vi "Graph.vi"(8 "error in (no error)":errorcluster, 10 "notifier out":refnum<notifier>, 11 "State in":T1={"State"=enum."Idle", "Start Time"=timestamp(0 s since 1904-01-01), "Current Time"=timestamp(0 s since 1904-01-01), "First Iteration"=FALSE, "Data"={"D-O State"=enum."Off"}, "Process Name"="", "Output Error"=FALSE, "Log Started"=FALSE, "Cycle Period"=50.0, "Configuration"={"Valve Settings"={"D-O Settings"={"DAQmx Task Name"="", "Output Channel"=0, "Output Channel Names"=[]}, "VICI Electronic Actuator"={"VISA resource name"="", "Mode"=enum."Two Positions With Stops", "Simulated"=FALSE}}, "Valve Type"=enum."Digital Output Valve", "Time On (Sec)"=0.0, "Time Off (Sec)"=0.0, "Run?"=FALSE}} {"Configuration"."Valve Settings"."D-O Settings"."Output Channel" items=["Choose a Channel"]}) -> (0 "error out":errorcluster, 3 "State out":T1={"State"=enum."Idle", "Start Time"=timestamp(0 s since 1904-01-01), "Current Time"=timestamp(0 s since 1904-01-01), "First Iteration"=FALSE, "Data"={"D-O State"=enum."Off"}, "Process Name"="", "Output Error"=FALSE, "Log Started"=FALSE, "Cycle Period"=50.0, "Configuration"={"Valve Settings"={"D-O Settings"={"DAQmx Task Name"="", "Output Channel"=0, "Output Channel Names"=[]}, "VICI Electronic Actuator"={"VISA resource name"="", "Mode"=enum."Two Positions With Stops", "Simulated"=FALSE}}, "Valve Type"=enum."Digital Output Valve", "Time On (Sec)"=0.0, "Time Off (Sec)"=0.0, "Run?"=FALSE}} {"Configuration"."Valve Settings"."D-O Settings"."Output Channel" items=["Choose a Channel"]})   [LabVIEW 2018, in "D-O Module.lvlib" / "D-O Module Engine.lvlib"]
uses:
  D-O Module Engine.lvlib
  State Cluster.ctl
  State Enum.ctl
  Valve Clusters.ctl
  D-O Module Settings Cluster.ctl
  D-O Device Settings Cluster.ctl
  VICI Electronic Actuator/VICI Electronic Actuator Settings.ctl
  D-O Module.lvlib
  DIO Valve/VICI Electronic Actuator.lvlib
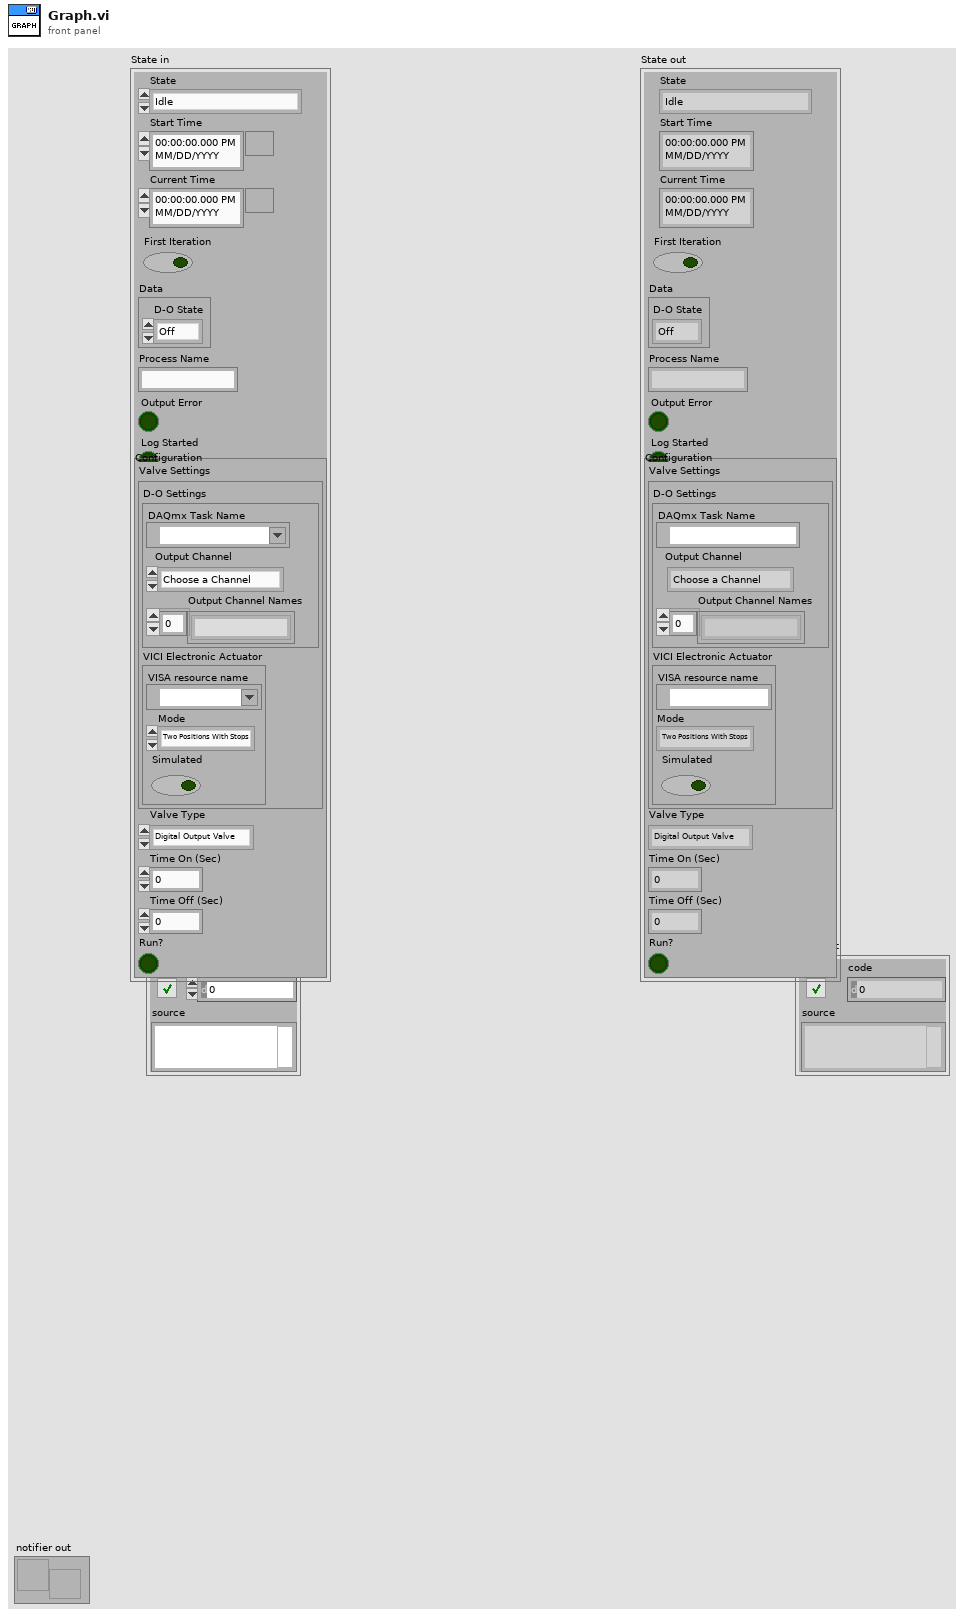
[diagram p1: front panel]
types:
  T1 = typedef "D-O Module.lvlib/D-O Module Engine.lvlib/State Cluster.ctl" = cluster{"State":T2, "Start Time":timestamp, "Current Time":timestamp, "First Iteration":bool, "Data":cluster{"D-O State":enum16{"Off", "On", "Not Initialized"}}, "Process Name":string, "Output Error":bool, "Log Started":bool, "Cycle Period":dbl, "Configuration":T3}
  T2 = typedef "D-O Module.lvlib/D-O Module Engine.lvlib/State Enum.ctl" = enum16{"Measuring", "Idle", "Paused"}
  T3 = typedef "D-O Module.lvlib/Valve Clusters.ctl" = cluster{"Valve Settings":T4, "Valve Type":enum16{"Default", "Digital Output Valve", "VICI Electronic Actuator"}, "Time On (Sec)":dbl, "Time Off (Sec)":dbl, "Run?":bool}
  T4 = typedef "D-O Module.lvlib/D-O Module Settings Cluster.ctl" = cluster{"D-O Settings":T5, "VICI Electronic Actuator":T6}
  T5 = typedef "D-O Module.lvlib/D-O Device Settings Cluster.ctl" = cluster{"DAQmx Task Name":refnum<k21>, "Output Channel":u16, "Output Channel Names":string[]}
  T6 = typedef "VICI Electronic Actuator.lvlib/VICI Electronic Actuator Settings.ctl" = cluster{"VISA resource name":refnum<visa-resource-name>, "Mode":enum16{"Two Positions With Stops", "Two Positions Without Stops", "Mutiposition"}, "Simulated":bool}
  T7 = cluster{"D-O State":enum16{"Off", "On", "Not Initialized"}}
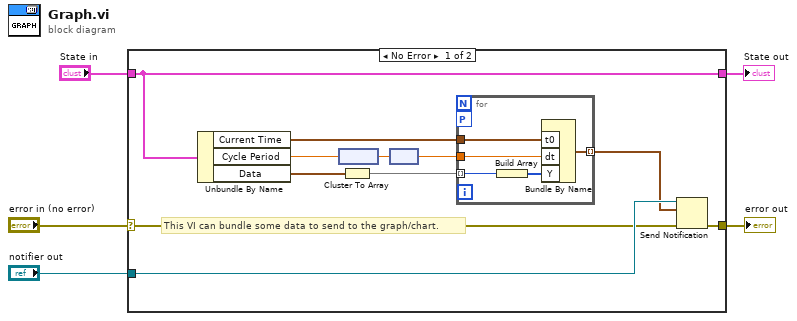
[diagram p0: block diagram]
diagram:
  n1 = case shown="No Error" "error in (no error)" {
    selector: "error in (no error)" -> [w13 w23]
    tunnel: [w12 w23] -> w4
    tunnel: "State in" -> [w16 w22]
    tunnel: [w16 w22] -> w2
    tunnel: "notifier out" -> [w14 _]
    frame No Error {
      # "This VI can bundle some data to send to the graph/chart."
      n2 = Unbundle By Name(w16) -> ("Current Time"=w11:timestamp, "Cycle Period"=w10:dbl, "Data"=w15:T7)
      n3 = node(w10) -> (w9:dbl[unit])
      n4 = Cluster To Array(cluster=w15) -> (array=w7:enum16{"Off", "On", "Not Initialized"}[])
      n5 = node(w9) -> (w8:dbl)
      n6 = for {
        tunnel: w11 -> [w21]
        tunnel: w8 -> [w20]
        tunnel: w7 -> [w19] mode=indexing
        tunnel: [w17] -> w6 mode=indexing
        workers-P: _ -> [_]
        n7 = Build Array(w19) -> (w18:enum16{"Off", "On", "Not Initialized"}[])
        n8 = Bundle By Name("t0"=w21, "dt"=w20, "Y"=w18) -> (w17:waveform(u16))  [unwired: 1 in]
      }
      n9 = Send Notification(notification=w6, notifier=w14, error in (no error)=w13) -> (error out=w12:errorcluster)  [unwired: 1 out]
    }
    frame Error {
    }
  }
  "error out" <- w4
  "State out" <- w2
